vi "Generate csproj from XML.vi"(7 "CD Root Folder Path":path, 8 "error in":errorcluster, 11 "XML File Path":path) -> (0 "error out":errorcluster, 3 "csproj Path":path, 5 "CD Gen code folder":path)   [LabVIEW 2026, in "NIVS_CDEW_MetaDataObj.lvclass"]
uses:
  NIVS_CDEW_MetaDataObj.lvclass
  Types/Errors.ctl
  NIVS_CDEW_MetaDataObj.lvclass/NIVS_CDEW_MetaDataObj.ctl
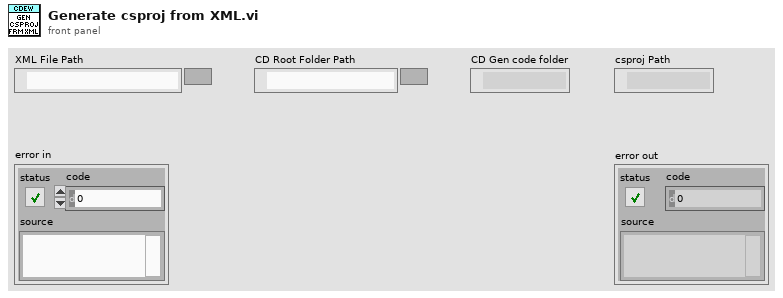
[diagram p1: front panel]
types:
  T1 = typedef "NIVS_CDEW_MetaDataObj.lvclass/Errors.ctl" = i32
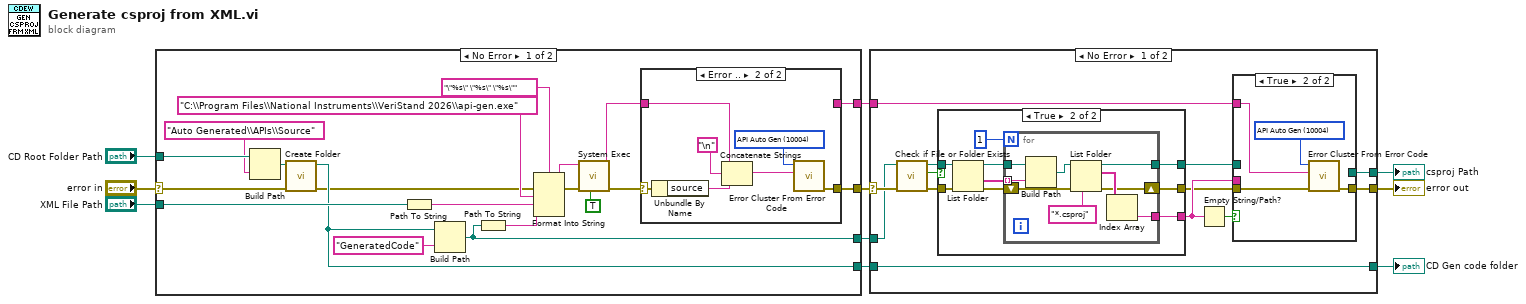
[diagram p0: block diagram]
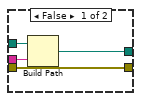
[diagram p3: hidden frame]
diagram:
  n1 = case shown="No Error" "error in" {
    selector: "error in" -> [w17 w40]
    tunnel: "XML File Path" -> [w24 _]
    tunnel: [w12 w40] -> w8
    tunnel: [w25 _] -> w6
    tunnel: "CD Root Folder Path" -> [w20 _]
    tunnel: [w11 _] -> w2
    tunnel: [w18 _] -> w1
    frame No Error {
      n2 = Build Path(base path=w20, name or relative path="Auto Generated\\APIs\\Source") -> (appended path=w21:path)
      n3 = call "Create Folder.vi"("error in"=w17, "Folder Path"=w21) -> ("error out"=w16:errorcluster, "Folder Path Out"=w18:path)  [unwired: 8 in]
      n4 = Path To String(path=w24) -> (string=w29:string)
      n5 = Build Path(base path=w18, name or relative path="GeneratedCode" ("format string")) -> (appended path=w25:path)
      n6 = Path To String(path=w25) -> (string=w26:string)
      n7 = Format Into String(format string="\"%s\" \"%s\" \"%s\"", error in=w16, "C:\\Program Files\\National Instruments\\VeriStand 2026\\api-gen.exe", w29, w26) -> (resulting string=w28:string, error out=w15:errorcluster)  [unwired: 1 in]
      n8 = call <vilib>:"System Exec.vi"("run minimized? (F)"=TRUE, "error in (no error)"=w15, "command line"=w28) -> ("error out"=w14:errorcluster, "standard output"=w13:string)  [unwired: 5 in, 2 out]
      n9 = case shown="Error .." w14 {
        selector: w14 -> [w31 w37]
        tunnel: w13 -> [w32 w38]
        tunnel: [w31 w39] -> w12
        tunnel: [w32 _] -> w11
        frame No Error {
        }
        frame Error {
          w33 = T1 10004 items=["Invalid XML File"=10001, "Missing File/Folder"=10002, "Duplicate CD in Root"=10003, "API Auto Gen"=10004, "Build APIs"=10005, "Clusters Auto Gen"=10006, "Create LV Projects"=10007] ("Errors")
          n10 = Unbundle By Name(w37) -> ("source"=w36:string)
          n11 = Concatenate Strings(w38, "\n", w36) -> (w34:string)
          n12 = call <vilib>:"Error Cluster From Error Code.vi"("error message (\"\")"=w34, "error code (0)"=w33) -> ("error out"=w39:errorcluster)  [unwired: 7 in]
        }
      }
    }
    frame Error {
    }
  }
  n13 = case shown="No Error" w8 {
    selector: w8 -> [w46 w81]
    tunnel: [w52 w81] -> w7
    tunnel: w6 -> [w44 _]
    tunnel: [w49 _] -> w5
    tunnel: [w47 _] -> w4
    tunnel: w2 -> [w48 _]
    tunnel: w1 -> [w47 _]
    frame No Error {
      n14 = call <vilib>:"Check if File or Folder Exists.vi"("error in (no error)"=w46, "path"=w44) -> ("error out"=w45:errorcluster, "file or folder exists?"=w42:bool, "dup path"=w43:path)  [unwired: 7 in]
      n15 = case shown="True" w42 {
        tunnel: [_ w60] -> w51
        tunnel: [_ w59] -> w50
        tunnel: w45 -> [w54 w58]
        tunnel: w43 -> [_ w57]
        tunnel: [w54 w55] -> w41
        frame False {
        }
        frame True {
          n16 = List Folder(path=w57, error in=w58) -> (path out=w63:path, folder names=w61:string[], error out=w56:errorcluster)  [unwired: 2 in, 1 out]
          n17 = for {
            N: 1 -> [_]
            tunnel: w63 -> [w72]
            tunnel: w61 -> [w71] mode=indexing
            tunnel: [w67] -> w60
            tunnel: [w66] -> w59
            shift-right: [w64] -> w55
            shift-left: w56 -> [w65]
            n18 = Build Path(base path=w72, name or relative path=w71) -> (appended path=w70:path)
            n19 = List Folder(path=w70, pattern="*.csproj", error in=w65) -> (path out=w66:path, filenames=w68:string[], error out=w64:errorcluster)  [unwired: 1 in, 1 out]
            n20 = Index Array(array=w68) -> (element=w67:string)  [unwired: 1 in]
          }
        }
      }
      n21 = Empty String/Path?(string/path=w51) -> (empty?=w53:bool)
      n22 = case shown="True" w53 {
        tunnel: w41 -> [w76 w79]
        tunnel: [w76 w80] -> w52
        tunnel: w51 -> [w74 _]
        tunnel: w50 -> [w75 _]
        tunnel: [w73 _] -> w49
        tunnel: w48 -> [_ w78]
        frame False {
          n23 = Build Path(base path=w75, name or relative path=w74) -> (appended path=w73:path)
        }
        frame True {
          w77 = T1 10004 items=["Invalid XML File"=10001, "Missing File/Folder"=10002, "Duplicate CD in Root"=10003, "API Auto Gen"=10004, "Build APIs"=10005, "Clusters Auto Gen"=10006, "Create LV Projects"=10007] ("Errors")
          n24 = call <vilib>:"Error Cluster From Error Code.vi"("error in (no error)"=w79, "error message (\"\")"=w78, "error code (0)"=w77) -> ("error out"=w80:errorcluster)  [unwired: 6 in]
        }
      }
    }
    frame Error {
    }
  }
  "error out" <- w7
  "csproj Path" <- w5
  "CD Gen code folder" <- w4
